vi "Cmd-Rec objectRepository.vi"(0 "command-recordset reference":T2, 1 "method":T3, 2 "occurrence":refnum<k4>, 5 "flags in":i32 format="%.0x", 7 "name in":string, 9 "classDataIn":T4, 11 "error in (no error)":errorcluster) -> (4 "command-recordset reference out":T2, 6 "flags out":i32 format="%.0x", 8 "name out":string, 10 "classDataOut":T4, 13 "stats":T1 {"time" format="%<%I:%M:%S%2u %p>T"}, 14 "[references out]":i32[](array[numeric]) format="%.0x", 15 "error out":errorcluster)   [LabVIEW 2012, in "NI_Database_API_64.lvlib"]
doc: "This VI manages objects of the <B>Command-Recordset</B> class.\n\n[GOOP 1.0/1.0]"
uses:
  NI_Database_API_64.lvlib
  Cmd-Rec Object Reference.ctl
  Cmd-Rec Data Members.ctl
  Recordset.llb/Rec ObjectReference.ctl
  Command.llb/Cmd ObjectReference.ctl
  <vilib>/Utility/_goopsup.llb/GOOP Object Repository Method.ctl
  <vilib>/Utility/_goopsup.llb/GOOP Object Repository Statistics.ctl
panel:
  in  "debugging":bool
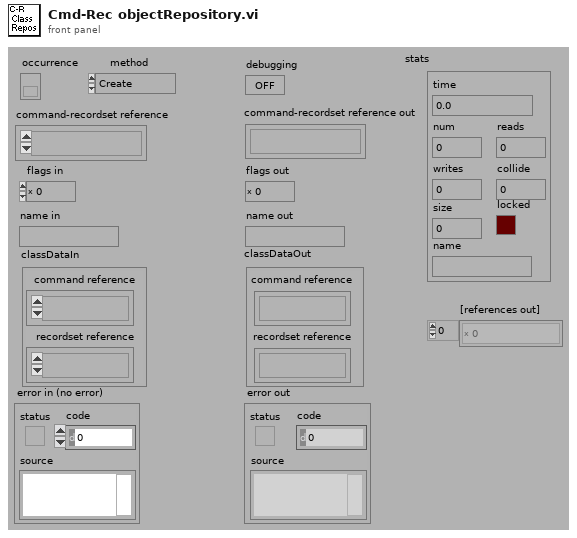
[diagram p1: front panel]
types:
  T1 = typedef "GOOP Object Repository Statistics.ctl" = cluster{"time":dbl, "num":u32, "reads":u32, "writes":u32, "collide":u32, "size":u32, "name":string, "locked":bool}
  T2 = typedef "NI_Database_API_64.lvlib/Cmd-Rec Object Reference.ctl" = refnum<k1>
  T3 = typedef "GOOP Object Repository Method.ctl" = enum16{"Create", "GetCopy", "GetModify", "Set", "Destroy", "Create Static", "Get All Refs", "Reset", "Get Statistics"}
  T4 = typedef "NI_Database_API_64.lvlib/Cmd-Rec Data Members.ctl" = cluster{"recordset reference":T5, "command reference":T6}
  T5 = typedef "NI_Database_API_64.lvlib/Rec ObjectReference.ctl" = refnum<k1>
  T6 = typedef "NI_Database_API_64.lvlib/Cmd ObjectReference.ctl" = refnum<k1>
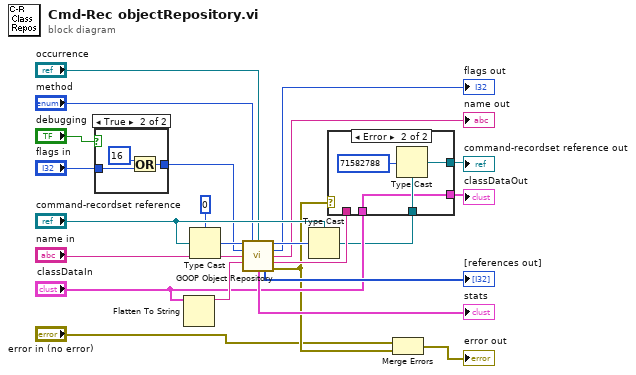
[diagram p0: block diagram]
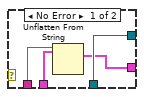
[diagram p2: hidden frame]
diagram:
  n1 = case shown="True" "debugging" {
    tunnel: "flags in" -> [w24 w27]
    tunnel: [w24 w26] -> w12
    frame False {
    }
    frame True {
      n2 = Or(x=16, y=w27) -> (x .or. y?=w26:i32)
    }
  }
  n3 = Flatten To String(anything="classDataIn") -> (data string=w16:string)  [unwired: 1 in, 4 out]
  n4 = Type Cast(type=0 ("object ref in"), x="command-recordset reference") -> (*(type *) &x=w21:i32)
  n5 = call <vilib>:"GOOP Object Repository.vi"("object ref in"=w21, "method"="method", "occurrence"="occurrence", "flags in"=w12, "name in"="name in", "object data in"=w16) -> ("object ref out"=w19:i32, "flags out"=→"flags out":i32, "name out"=→"name out":string, "object data out"=w7:string, "stats"=→"stats":T1, "[references out]"=→"[references out]":i32[], "error out"=w2:errorcluster)  [unwired: 1 in, 2 out]
  n6 = Type Cast(type="command-recordset reference", x=w19) -> (*(type *) &x=w5:T2)
  n7 = case shown="Error" w2 {
    tunnel: w5 -> [w31 w35]
    tunnel: [w31 w33] -> w4
    tunnel: w7 -> [w30 _]
    tunnel: "classDataIn" -> [w29 w32]
    tunnel: [w28 w32] -> w8
    frame No Error {
      n8 = Unflatten From String(type=w29, binary string=w30) -> (value=w28:T4)  [unwired: 1 in, 4 out]
    }
    frame Error {
      n9 = Type Cast(type=w35, x=71582788) -> (*(type *) &x=w33:T2)
    }
  }
  "command-recordset reference out" <- w4
  "classDataOut" <- w8
  n10 = Merge Errors("error in (no error)", w2) -> (→"error out":errorcluster)
